vi "niFPGA Discrete Control Filter_m.vi"   [LabVIEW 2017]
doc: "Applies a fifth-order low-pass integer FIR filter to the input data. The filter cut-off frequency is 1/10 of the sample frequency of the <B>input</B>. Use the Discrete Control Filter VI to filter measured values, such as the process variable, in control applications. The data type you wire to <B>input</B> determines the <B>output</B> data type."
uses:
  <vilib>/rvi/Analysis/common/FxpNativeNode/niFpgaFxpNative.xnode
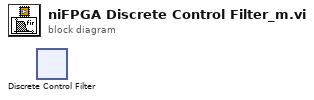
[diagram p0: block diagram]
diagram:
  n1 = xnode "Discrete Control Filter"() -> ()  [unwired: 2 in, 1 out]
